vi "Conversao_todos_e_link_CLP.vi"() -> ()   [LabVIEW 2019]
uses:
  padrao_UCM.004.EEL.0300_ENTRADA.ctl
  padrao_UCM.004.EEL.0300_SAIDA.ctl
  padrao_UCM.004.EEL.0200_ENTRADA.ctl
  padrao_UCM.004.EEL.0200_SAIDA.ctl
  padrao_INTERNO.ctl
  padrao_todos_os_dados_ENTRADA.ctl
  padrao_todos_os_dados_SAIDA.ctl
  <vilib>/Utility/config.llb/NI_LVConfig.lvlib
panel:
  out "INTERNO":T1
  out "UCM.004.EEL.0200_ENTRADA_engenharia":T2
  out "X33-2":i16
  out "GD-ST-ES":i16
  out "X31-16":bool
  out "X31-15":bool
  out "X31-14":bool
  out "X31-13":bool
  out "X31-12":bool
  out "X31-11":bool
  out "X31-10":bool
  out "SHD-ON-OFF":bool
  out "SHD-CV-002":bool
  out "SHD-CV-001":bool
  out "SKS-CV-006":bool
  out "SKS-CV-005":bool
  out "SKS-CV-004":bool
  out "SKS-CV-003":bool
  out "SKS-CV-002":bool
  out "SKS-CV-001":bool
  in  "SIT-PI-03":i16
  in  "SIT-PI-MS3":i16
  in  "SHD-PI-02":i16
  in  "SHD-PI-01":i16
  in  "X32-4":i16
  in  "SHD-TI-AMB":i16
  in  "SKS-LC-W":i16
  in  "SKS-LC-K":i16
  in  "X30-16":bool
  in  "X30-15":bool
  in  "X30-14":bool
  in  "X30-13":bool
  in  "X30-12":bool
  in  "X30-11":bool
  in  "X30-10":bool
  in  "X30-9":bool
  in  "X30-8":bool
  in  "SKS-MAX-K":bool
  in  "SKS-MIN-K":bool
  in  "SKS-MAX-W":bool
  in  "SKS-MIN-W":bool
  in  "SKS-LAH-K":bool
  in  "SKS-LAH-W":bool
  in  "SKS-LAH-S":bool
  out "UCM.004.EEL.0200_SAIDA(%)":T3
  out "UCM.004.EEL.0200_SAIDA(Puro)":T3
  out "UCM.004.EEL.0200_ENTRADA_puro":T2
  out "UCM.004.EEL.0300_SAIDA(%)":T4
  in  "SKM-FIC-COR-AR":dbl
  out "PID-INV-KF-GD":dbl
  out "PID-INV-KF-GI":dbl
  out "PID-INV-KF-GP":dbl
  out "PID-INV-WF-GD":dbl
  out "PID-INV-WF-GI":dbl
  out "PID-INV-WF-GP":dbl
  out "PID-FC-KF-GD":dbl
  out "PID-FC-KF-GI":dbl
  out "PID-FC-KF-GP":dbl
  out "PID-FC-WF-GD":dbl
  out "PID-FC-WF-GI":dbl
  out "PID-FC-WF-GP":dbl
  out "PID-FC-AR-GD":dbl
  out "PID-FC-AR-GI":dbl
  out "PID-FC-AR-GP":dbl
  out "PID-PC-TQ-GD":dbl
  out "PID-PC-TQ-GI":dbl
  out "PID-PC-TQ-GP":dbl
  out "SKM-FIC-COR-KF-MIN":dbl
  out "SKM-FIC-COR-KF-MAX":dbl
  out "SKM-FIC-COR-AR-MIN":dbl
  out "SKM-FIC-COR-AR-MAX":dbl
  out "SPW-WR-VEL":i32
  out "SPK-WR-VEL":i32
  out "PID-INC-KF-SP":i16
  out "PID-INC-WF-SP":i16
  out "PID-FC-KF-SP":i16
  out "PID-FC-WF-SP":i16
  out "PID-FC-AR-SP":i16
  out "PID-PC-TQ-SP":i16
  out "X33 14":i16
  out "X33 13":i16
  out "X33 12":i16
  out "X33 11":i16
  out "X33 10":i16
  out "X33 9":i16
  out "X33 8":i16
  out "X33 7":i16
  out "X33 6":i16
  out "X33 5":i16
  out "SKM-FC-KF":i16
  out "SKM-FC-WF":i16
  out "SKM-FC-AR":i16
  out "SKM-PC-TQ":i16
  out "UCM.004.EEL.0300_SAIDA(Puro)":T4
  out "SPW-WR-OFF":bool
  out "SPK-WR-OFF":bool
  out "SPW-WR-ON":bool
  out "SPK-WR-ON":bool
  out "PID-SA-AR-COR":bool
  out "PID-SA-KF-INV":bool
  out "PID-SA-WF-INV":bool
  out "PID-KF-ON":bool
  out "PID-WF-ON":bool
  out "PID-FC-AR-ON":bool
  out "PID-PC-TQ-ON":bool
  out "X31-32":bool
  out "X31-31":bool
  out "X31-30":bool
  out "X31-29":bool
  out "X31-28":bool
  out "X31-27":bool
  out "SKI-CV-BY2":bool
  out "SKI-CV-ST":bool
  out "SKI-CV-WF-BY1":bool
  out "SKI-CV-WF-ST":bool
  out "SKI-CV-KF-BY1":bool
  out "SKI-CV-KF-ST":bool
  out "SKI-CV-AR":bool
  out "SKM-CV-JMP":bool
  out "SKM-CV-COR":bool
  out "SKM-CV-LAM":bool
  out "SPW-CV-008":bool
  out "SPW-CV-007":bool
  out "SPW-CV-006":bool
  out "SPW-CV-005":bool
  out "SPW-CV-004":bool
  out "SPW-CV-003":bool
  out "SPW-CV-002":bool
  out "SPW-CV-001":bool
  out "SPK-CV-008":bool
  out "SPK-CV-007":bool
  out "SPK-CV-006":bool
  out "SPK-CV-005":bool
  out "SPK-CV-004":bool
  out "SPK-CV-003":bool
  out "SPK-CV-002":bool
  out "SPK-CV-001":bool
  in  "SPW-RD-CRT":dbl
  in  "SPK-RD-CRT":dbl
  in  "SKM-DEN-COR-AR":dbl
  in  "SKM-TI-COR-AR":dbl
  in  "SKM-FIC-COR-KF":dbl
  in  "SKM-DEN-COR-KF":dbl
  in  "SKM-TI-COR-KF":dbl
  in  "SPW-RD-TU":i32
  in  "SPK-RD-TU":i32
  in  "SPW-RD-IA":i32
  in  "SPK-RD-IA":i32
  in  "SPW-RD-VEL":i32
  in  "SPK-RD-VEL":i32
  in  "SPW-RD-ST":i32
  in  "SPK-RD-ST":i32
  in  "X32 24":i16
  in  "X32 23":i16
  in  "X32 22":i16
  in  "X32 21":i16
  in  "X32 20":i16
  in  "X32 19":i16
  in  "X32 18":i16
  in  "X32 17":i16
  in  "X32 16":i16
  in  "SPK-PD-P":i16
  in  "SPW-PD-P":i16
  in  "SKM-TI-KF":i16
  in  "SIT-PI-MS2":i16
  in  "SIT-PI-MS1":i16
  in  "SKI-PD-ST":i16
  in  "SIT-PI-001":i16
  in  "SKM-FIM-WF":i16
  in  "SKM-TI-WF":i16
  in  "SKM-PD-LAM":i16
  in  "SKM-TI-LAM":i16
  in  "SKM-PA-LAM":i16
  in  "SKM-TI-TQ":i16
  in  "SKM-PA-TQ":i16
  in  "SKM-PA-BAR":i16
  in  "SPW-RD-FLL":bool
  in  "SPW-RD-VVT":bool
  in  "SPW-RD-ALR":bool
  in  "SPK-RD-FLL":bool
  in  "SPK-RD-VVT":bool
  in  "SPK-RD-ALR":bool
  in  "X30 16":bool
  in  "X30 15":bool
  in  "X30 14":bool
  in  "X30 13":bool
  in  "X30 12":bool
  in  "X30 11":bool
  in  "X30 10":bool
  in  "X30 9":bool
  in  "X30 8":bool
  in  "X30 7":bool
  in  "X30 6":bool
  in  "X30 5":bool
  in  "X30 4":bool
  in  "X30 3":bool
  in  "X30 2":bool
  in  "X30 1":bool
  out "UCM.004.EEL.0300_ENTRADA_engenharia":T5
  out "UCM.004.EEL.0300_ENTRADA_puro":T5
  in  "stop":bool
  # "DADOS INTERNO"
  # "LEITURA\nENTRADA"
  # "ESCRITA\nSAIDA"
  # "0300"
  # "0300"
  # "0200"
  # "0200"
  # "PURO"
  # "ENGENHARIA"
  # "PURO"
  # "ENGENHARIA"
  # "(%)"
  # "PURO"
  # "(%)"
  # "PURO"
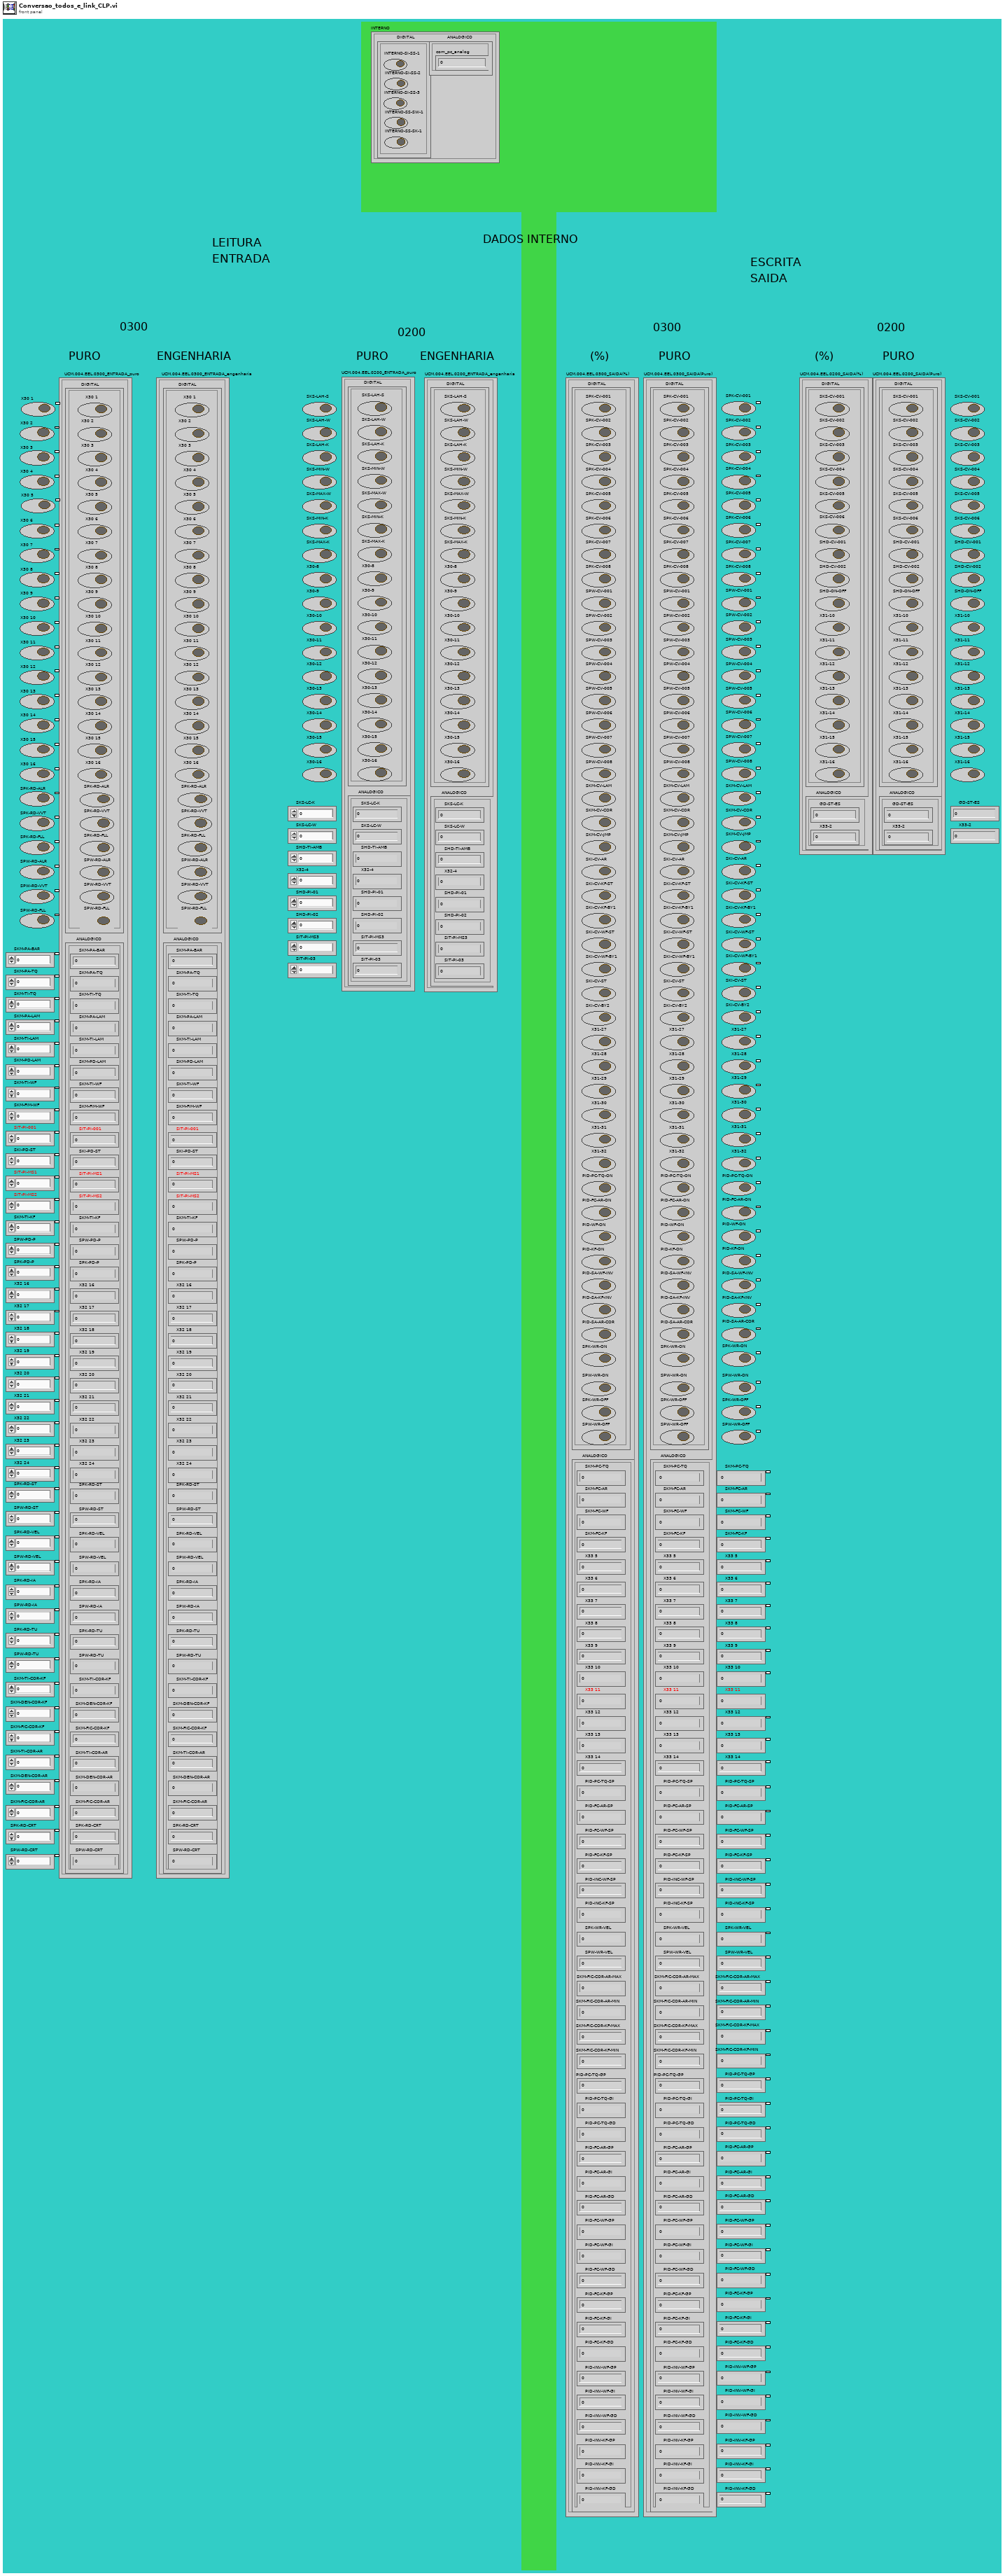
[diagram p1: front panel]
types:
  T1 = typedef "padrao_INTERNO.ctl" = cluster{"DIGITAL":cluster{"INTERNO-SI-SS-1":bool, "INTERNO-SI-SS-2":bool, "INTERNO-SI-SS-3":bool, "INTERNO-SS-SW-1":bool, "INTERNO-SS-SK-1":bool}, "ANALOGICO":cluster{"com_pc_analog":dbl}}
  T2 = typedef "padrao_UCM.004.EEL.0200_ENTRADA.ctl" = cluster{"DIGITAL":cluster{"SKS-LAH-S":bool, "SKS-LAH-W":bool, "SKS-LAH-K":bool, "SKS-MIN-W":bool, "SKS-MAX-W":bool, "SKS-MIN-K":bool, "SKS-MAX-K":bool, "X30-8":bool, "X30-9":bool, "X30-10":bool, "X30-11":bool, "X30-12":bool, "X30-13":bool, "X30-14":bool, "X30-15":bool, "X30-16":bool}, "ANALOGICO":cluster{"SKS-LC-K":i16, "SKS-LC-W":i16, "SHD-TI-AMB":i16, "X32-4":i16, "SHD-PI-01":i16, "SHD-PI-02":i16, "SIT-PI-MS3":i16, "SIT-PI-03":i16}}
  T3 = typedef "padrao_UCM.004.EEL.0200_SAIDA.ctl" = cluster{"DIGITAL":cluster{"SKS-CV-001":bool, "SKS-CV-002":bool, "SKS-CV-003":bool, "SKS-CV-004":bool, "SKS-CV-005":bool, "SKS-CV-006":bool, "SHD-CV-001":bool, "SHD-CV-002":bool, "SHD-ON-OFF":bool, "X31-10":bool, "X31-11":bool, "X31-12":bool, "X31-13":bool, "X31-14":bool, "X31-15":bool, "X31-16":bool}, "ANALOGICO":cluster{"GD-ST-ES":i16, "X33-2":i16}}
  T4 = typedef "padrao_UCM.004.EEL.0300_SAIDA.ctl" = cluster{"DIGITAL":cluster{"SPK-CV-001":bool, "SPK-CV-002":bool, "SPK-CV-003":bool, "SPK-CV-004":bool, "SPK-CV-005":bool, "SPK-CV-006":bool, "SPK-CV-007":bool, "SPK-CV-008":bool, "SPW-CV-001":bool, "SPW-CV-002":bool, "SPW-CV-003":bool, "SPW-CV-004":bool, "SPW-CV-005":bool, "SPW-CV-006":bool, "SPW-CV-007":bool, "SPW-CV-008":bool, "SKM-CV-LAM":bool, "SKM-CV-COR":bool, "SKM-CV-JMP":bool, "SKI-CV-AR":bool, "SKI-CV-KF-ST":bool, "SKI-CV-KF-BY1":bool, "SKI-CV-WF-ST":bool, "SKI-CV-WF-BY1":bool, "SKI-CV-ST":bool, "SKI-CV-BY2":bool, "X31-27":bool, "X31-28":bool, "X31-29":bool, "X31-30":bool, "X31-31":bool, "X31-32":bool, "PID-PC-TQ-ON":bool, "PID-FC-AR-ON":bool, "PID-WF-ON":bool, "PID-KF-ON":bool, "PID-SA-WF-INV":bool, "PID-SA-KF-INV":bool, "PID-SA-AR-COR":bool, "SPK-WR-ON":bool, "SPW-WR-ON":bool, "SPK-WR-OFF":bool, "SPW-WR-OFF":bool}, "ANALOGICO":cluster{"SKM-PC-TQ":i16, "SKM-FC-AR":i16, "SKM-FC-WF":i16, "SKM-FC-KF":i16, "X33 5":i16, "X33 6":i16, "X33 7":i16, "X33 8":i16, "X33 9":i16, "X33 10":i16, "X33 11":i16, "X33 12":i16, "X33 13":i16, "X33 14":i16, "PID-PC-TQ-SP":i16, "PID-FC-AR-SP":i16, "PID-FC-WF-SP":i16, "PID-FC-KF-SP":i16, "PID-INC-WF-SP":i16, "PID-INC-KF-SP":i16, "SPK-WR-VEL":i32, "SPW-WR-VEL":i32, "SKM-FIC-COR-AR-MAX":dbl, "SKM-FIC-COR-AR-MIN":dbl, "SKM-FIC-COR-KF-MAX":dbl, "SKM-FIC-COR-KF-MIN":dbl, "PID-PC-TQ-GP":dbl, "PID-PC-TQ-GI":dbl, "PID-PC-TQ-GD":dbl, "PID-FC-AR-GP":dbl, "PID-FC-AR-GI":dbl, "PID-FC-AR-GD":dbl, "PID-FC-WF-GP":dbl, "PID-FC-WF-GI":dbl, "PID-FC-WF-GD":dbl, "PID-FC-KF-GP":dbl, "PID-FC-KF-GI":dbl, "PID-FC-KF-GD":dbl, "PID-INV-WF-GP":dbl, "PID-INV-WF-GI":dbl, "PID-INV-WF-GD":dbl, "PID-INV-KF-GP":dbl, "PID-INV-KF-GI":dbl, "PID-INV-KF-GD":dbl}}
  T5 = typedef "padrao_UCM.004.EEL.0300_ENTRADA.ctl" = cluster{"DIGITAL":cluster{"X30 1":bool, "X30 2":bool, "X30 3":bool, "X30 4":bool, "X30 5":bool, "X30 6":bool, "X30 7":bool, "X30 8":bool, "X30 9":bool, "X30 10":bool, "X30 11":bool, "X30 12":bool, "X30 13":bool, "X30 14":bool, "X30 15":bool, "X30 16":bool, "SPK-RD-ALR":bool, "SPK-RD-VVT":bool, "SPK-RD-FLL":bool, "SPW-RD-ALR":bool, "SPW-RD-VVT":bool, "SPW-RD-FLL":bool}, "ANALOGICO":cluster{"SKM-PA-BAR":i16, "SKM-PA-TQ":i16, "SKM-TI-TQ":i16, "SKM-PA-LAM":i16, "SKM-TI-LAM":i16, "SKM-PD-LAM":i16, "SKM-TI-WF":i16, "SKM-FIM-WF":i16, "SIT-PI-001":i16, "SKI-PD-ST":i16, "SIT-PI-MS1":i16, "SIT-PI-MS2":i16, "SKM-TI-KF":i16, "SPW-PD-P":i16, "SPK-PD-P":i16, "X32 16 ":i16, "X32 17":i16, "X32 18":i16, "X32 19":i16, "X32 20":i16, "X32 21":i16, "X32 22":i16, "X32 23":i16, "X32 24":i16, "SPK-RD-ST":i32, "SPW-RD-ST":i32, "SPK-RD-VEL":i32, "SPW-RD-VEL":i32, "SPK-RD-IA":i32, "SPW-RD-IA":i32, "SPK-RD-TU":i32, "SPW-RD-TU":i32, "SKM-TI-COR-KF":dbl, "SKM-DEN-COR-KF":dbl, "SKM-FIC-COR-KF":dbl, "SKM-TI-COR-AR":dbl, "SKM-DEN-COR-AR":dbl, "SPK-RD-CRT":dbl, "SPW-RD-CRT":dbl, "SKM-FIC-COR-AR":dbl}}
  T6 = typedef "padrao_todos_os_dados_SAIDA.ctl" = cluster{"UCM.004.EEL.0300_SAIDA":T4, "UCM.004.EEL.0200_SAIDA":T3, "INTERNO":T1}
  T7 = typedef "padrao_todos_os_dados_ENTRADA.ctl" = cluster{"UCM.004.EEL.0300_ENTRADA":T5, "UCM.004.EEL.0200_ENTRADA":T2, "INTERNO":T1}
  T8 = typedef "NI_LVConfig.lvlib/Config Data RefNum.ctl" = refnum<k1>
  T9 = typedef "padrao_array_cluster_calibracao.ctl" = cluster{"TAG":string, "Minimo":dbl, "Fabricante":string, "Maximo":dbl, "remover_dipositvo":bool, "Modelo":string, "Numero de Serie":string}[]
  T10 = cluster{"SKS-CV-001":bool, "SKS-CV-002":bool, "SKS-CV-003":bool, "SKS-CV-004":bool, "SKS-CV-005":bool, "SKS-CV-006":bool, "SHD-CV-001":bool, "SHD-CV-002":bool, "SHD-ON-OFF":bool, "X31-10":bool, "X31-11":bool, "X31-12":bool, "X31-13":bool, "X31-14":bool, "X31-15":bool, "X31-16":bool}
  T11 = cluster{"SPK-CV-001":bool, "SPK-CV-002":bool, "SPK-CV-003":bool, "SPK-CV-004":bool, "SPK-CV-005":bool, "SPK-CV-006":bool, "SPK-CV-007":bool, "SPK-CV-008":bool, "SPW-CV-001":bool, "SPW-CV-002":bool, "SPW-CV-003":bool, "SPW-CV-004":bool, "SPW-CV-005":bool, "SPW-CV-006":bool, "SPW-CV-007":bool, "SPW-CV-008":bool, "SKM-CV-LAM":bool, "SKM-CV-COR":bool, "SKM-CV-JMP":bool, "SKI-CV-AR":bool, "SKI-CV-KF-ST":bool, "SKI-CV-KF-BY1":bool, "SKI-CV-WF-ST":bool, "SKI-CV-WF-BY1":bool, "SKI-CV-ST":bool, "SKI-CV-BY2":bool, "X31-27":bool, "X31-28":bool, "X31-29":bool, "X31-30":bool, "X31-31":bool, "X31-32":bool, "PID-PC-TQ-ON":bool, "PID-FC-AR-ON":bool, "PID-WF-ON":bool, "PID-KF-ON":bool, "PID-SA-WF-INV":bool, "PID-SA-KF-INV":bool, "PID-SA-AR-COR":bool, "SPK-WR-ON":bool, "SPW-WR-ON":bool, "SPK-WR-OFF":bool, "SPW-WR-OFF":bool}
  T12 = cluster{"SKM-PC-TQ":i16, "SKM-FC-AR":i16, "SKM-FC-WF":i16, "SKM-FC-KF":i16, "X33 5":i16, "X33 6":i16, "X33 7":i16, "X33 8":i16, "X33 9":i16, "X33 10":i16, "X33 11":i16, "X33 12":i16, "X33 13":i16, "X33 14":i16, "PID-PC-TQ-SP":i16, "PID-FC-AR-SP":i16, "PID-FC-WF-SP":i16, "PID-FC-KF-SP":i16, "PID-INC-WF-SP":i16, "PID-INC-KF-SP":i16, "SPK-WR-VEL":i32, "SPW-WR-VEL":i32, "SKM-FIC-COR-AR-MAX":dbl, "SKM-FIC-COR-AR-MIN":dbl, "SKM-FIC-COR-KF-MAX":dbl, "SKM-FIC-COR-KF-MIN":dbl, "PID-PC-TQ-GP":dbl, "PID-PC-TQ-GI":dbl, "PID-PC-TQ-GD":dbl, "PID-FC-AR-GP":dbl, "PID-FC-AR-GI":dbl, "PID-FC-AR-GD":dbl, "PID-FC-WF-GP":dbl, "PID-FC-WF-GI":dbl, "PID-FC-WF-GD":dbl, "PID-FC-KF-GP":dbl, "PID-FC-KF-GI":dbl, "PID-FC-KF-GD":dbl, "PID-INV-WF-GP":dbl, "PID-INV-WF-GI":dbl, "PID-INV-WF-GD":dbl, "PID-INV-KF-GP":dbl, "PID-INV-KF-GI":dbl, "PID-INV-KF-GD":dbl}
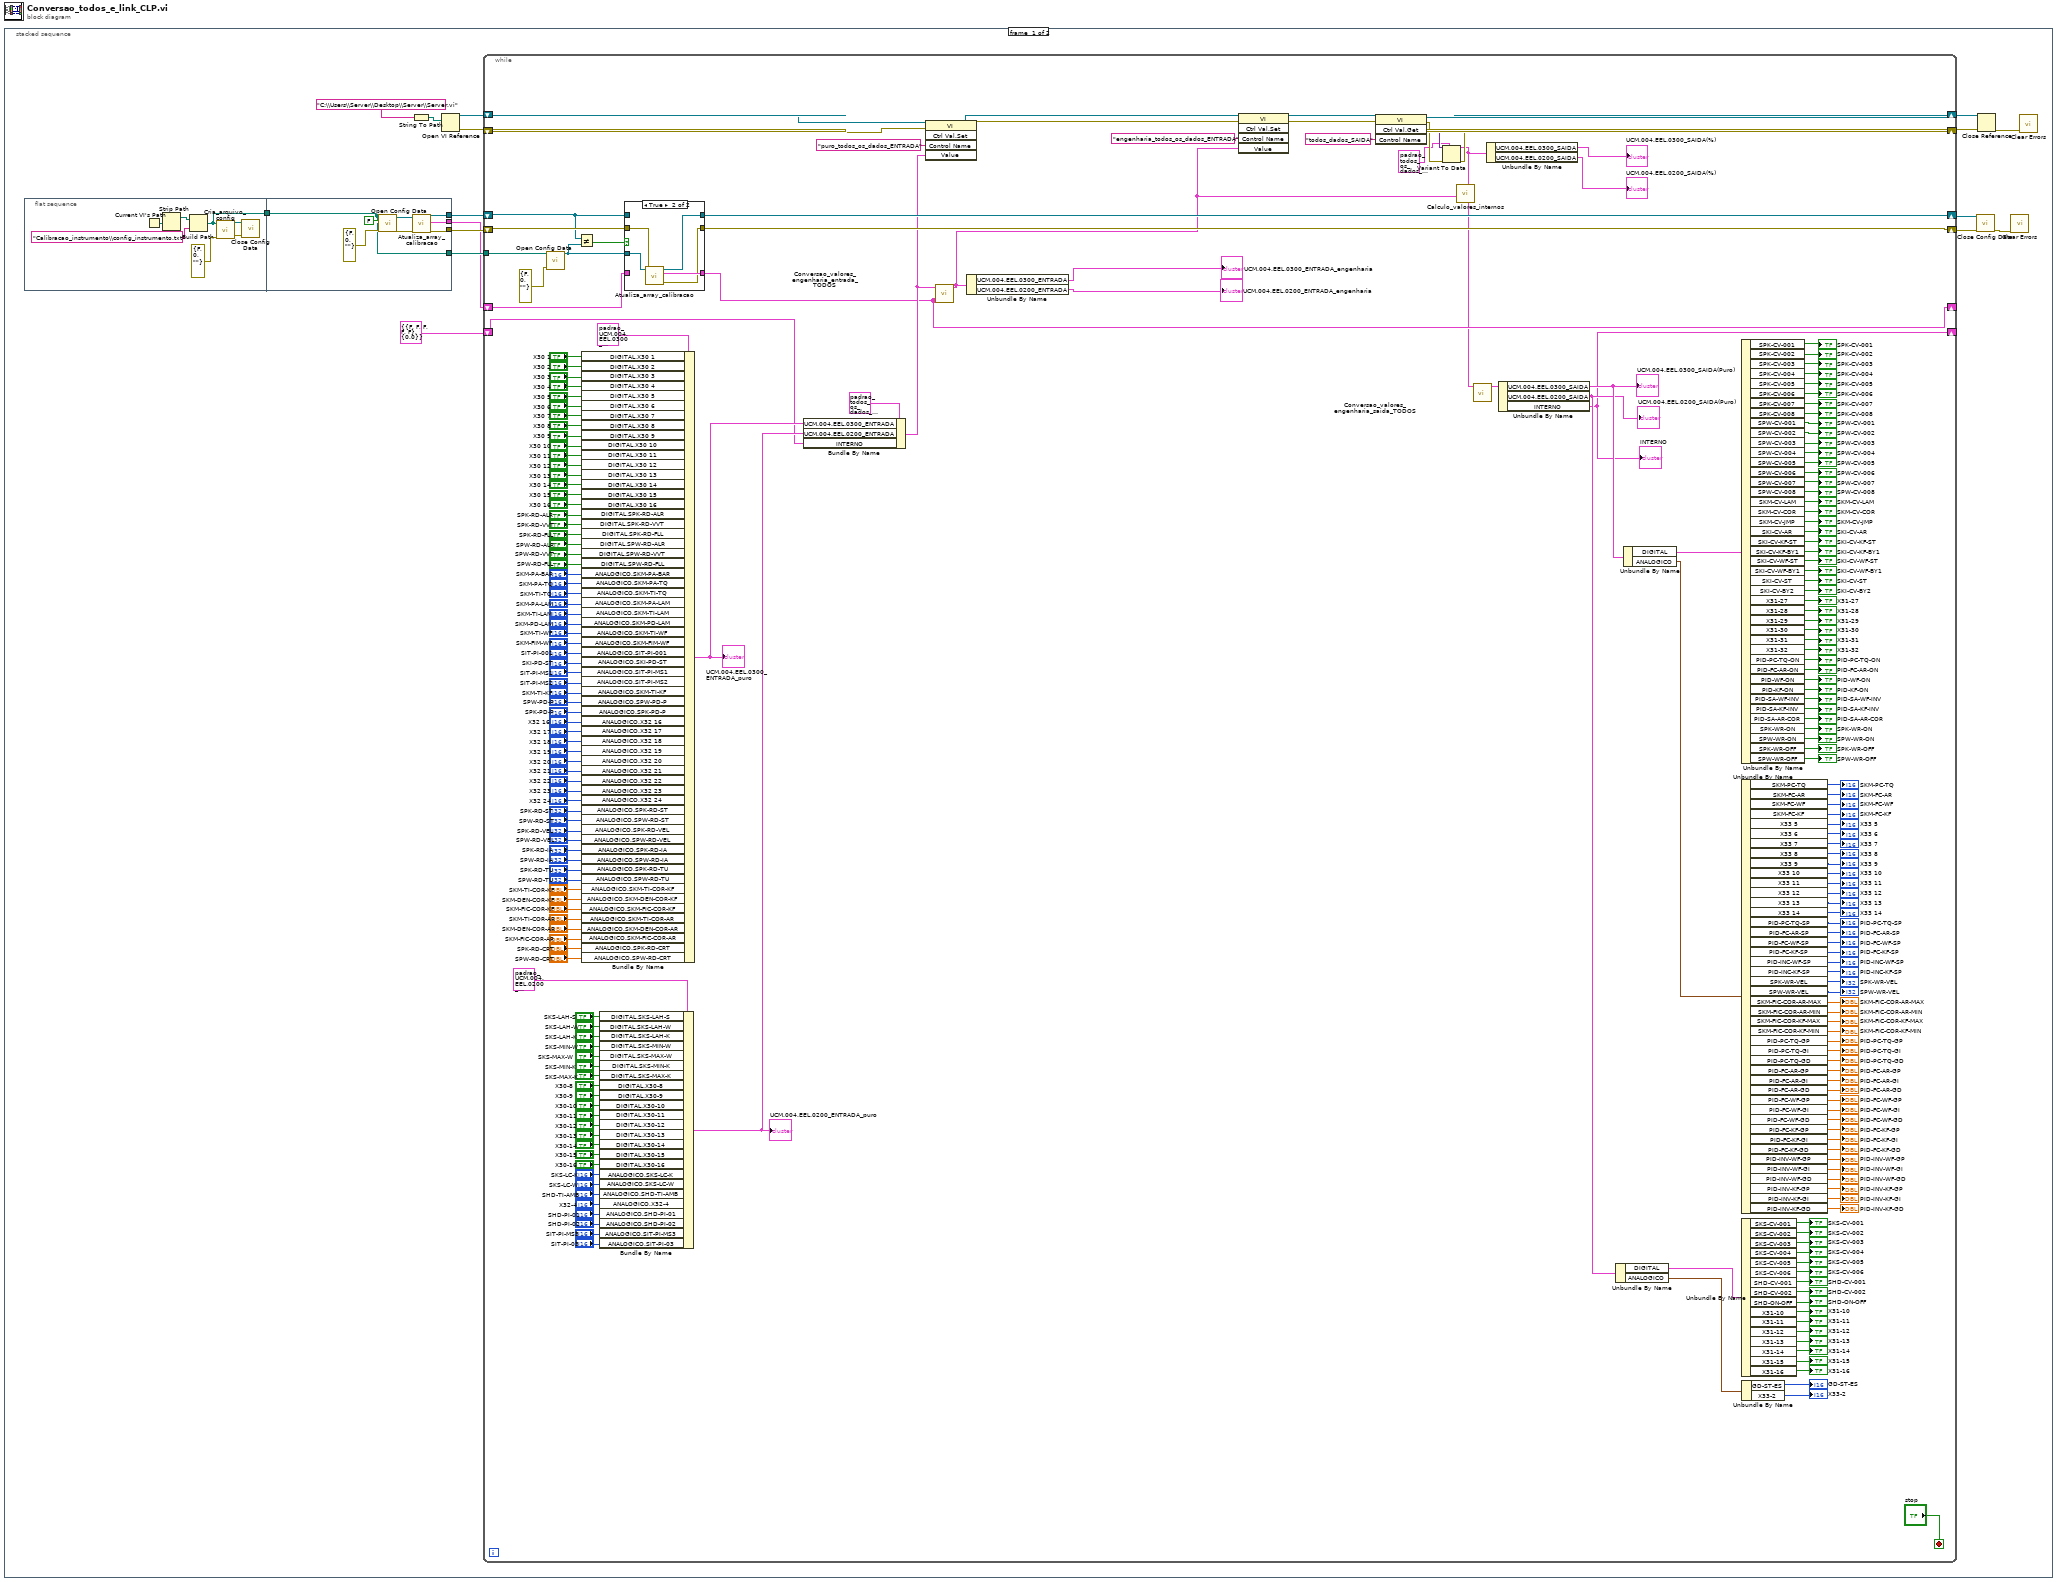
[diagram p0: block diagram]
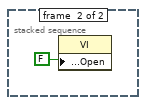
[diagram p3: hidden frame]
diagram:
  n1 = stacked-sequence {
    frame #0 {
      n2 = flat-sequence {
        tunnel: [w17] -> w6
        tunnel: w6 -> [w29]
        tunnel: [w28] -> w5
        tunnel: [w25] -> w4
        tunnel: [w29] -> w3
        tunnel: [w24] -> w2
        frame #0 {
          n3 = Current VI's Path() -> (path=w21:path)
          n4 = Strip Path(path=w21) -> (stripped path=w23:path)  [unwired: 1 out]
          n5 = Build Path(base path=w23, name or relative path="Calibracao_instrumento\\config_instrumento.txt") -> (appended path=w17:path)
          n6 = call "Cria_arquivo_config.vi"("error in (no error)"=errorcluster {"status"=FALSE, "code"=0, "source"=""}, "refnum in"=w17) -> ("error out"=w18:errorcluster, "refnum"=w19:T8)  [unwired: 8 in]
          n7 = call <vilib>:"Close Config Data.vi"("error in (no error)"=w18, "refnum"=w19) -> ()  [unwired: 8 in, 2 out]
        }
        frame #1 {
          n8 = call <vilib>:"Open Config Data.vi"("error in (no error)"=errorcluster {"status"=FALSE, "code"=0, "source"=""}, "create file if necessary (T)"=FALSE, "configuration file path"=w29) -> ("error out"=w26:errorcluster, "refnum"=w27:T8)  [unwired: 6 in, 1 out]
          n9 = call "Atualiza_array_calibracao.vi"("error in (no error)"=w26, "refnum"=w27) -> ("error out"=w25:errorcluster, "Instrumentos"=w24:T9, "refnum out"=w28:T8)  [unwired: 7 in]
        }
      }
      n10 = String To Path(string="C:\\Users\\Server\\Desktop\\Server\\Server.vi") -> (path=w15:path)
      n11 = Open VI Reference(vi path=w15) -> (vi reference=w13:refnum<vi>, error out=w14:errorcluster)  [unwired: 5 in]
      n12 = while {
        shift-right: [w258] -> w12
        shift-left: w13 -> [w269]
        shift-right: [w254] -> w11
        shift-left: w14 -> [w268]
        shift-right: [w98] -> w9
        shift-left: w5 -> [w94]
        shift-right: [w97] -> w8
        shift-left: w4 -> [w99]
        tunnel: w3 -> [w96]
        shift-right: [w86] -> _
        shift-left: w2 -> [w91]
        shift-right: [w35] -> _
        shift-left: T1 {"DIGITAL"={"INTERNO-SI-SS-1"=FALSE, "INTERNO-SI-SS-2"=FALSE, "INTERNO-SI-SS-3"=FALSE, "INTERNO-SS-SW-1"=FALSE, "INTERNO-SS-SK-1"=FALSE}, "ANALOGICO"={"com_pc_analog"=0.0}} ("INTERNO(Entrada)") -> [w36]
        stop <- "stop" stop-if-true
        n13 = call <vilib>:"Open Config Data.vi"("error in (no error)"=errorcluster {"status"=FALSE, "code"=0, "source"=""}, "configuration file path"=w96) -> ("refnum"=w92:T8)  [unwired: 7 in, 2 out]
        n14 = Not Equal?(x=w94, y=w92) -> (x != y?=w93:bool)
        n15 = Bundle By Name(cluster=T5 {"DIGITAL"={"X30 1"=FALSE, "X30 2"=FALSE, "X30 3"=FALSE, "X30 4"=FALSE, "X30 5"=FALSE, "X30 6"=FALSE, "X30 7"=FALSE, "X30 8"=FALSE, "X30 9"=FALSE, "X30 10"=FALSE, "X30 11"=FALSE, "X30 12"=FALSE, "X30 13"=FALSE, "X30 14"=FALSE, "X30 15"=FALSE, "X30 16"=FALSE, "SPK-RD-ALR"=FALSE, "SPK-RD-VVT"=FALSE, "SPK-RD-FLL"=FALSE, "SPW-RD-ALR"=FALSE, "SPW-RD-VVT"=FALSE, "SPW-RD-FLL"=FALSE}, "ANALOGICO"={"SKM-PA-BAR"=0, "SKM-PA-TQ"=0, "SKM-TI-TQ"=0, "SKM-PA-LAM"=0, "SKM-TI-LAM"=0, "SKM-PD-LAM"=0, "SKM-TI-WF"=0, "SKM-FIM-WF"=0, "SIT-PI-001"=0, "SKI-PD-ST"=0, "SIT-PI-MS1"=0, "SIT-PI-MS2"=0, "SKM-TI-KF"=0, "SPW-PD-P"=0, "SPK-PD-P"=0, "X32 16 "=0, "X32 17"=0, "X32 18"=0, "X32 19"=0, "X32 20"=0, "X32 21"=0, "X32 22"=0, "X32 23"=0, "X32 24"=0, "SPK-RD-ST"=0, "SPW-RD-ST"=0, "SPK-RD-VEL"=0, "SPW-RD-VEL"=0, "SPK-RD-IA"=0, "SPW-RD-IA"=0, "SPK-RD-TU"=0, "SPW-RD-TU"=0, "SKM-TI-COR-KF"=0.0, "SKM-DEN-COR-KF"=0.0, "SKM-FIC-COR-KF"=0.0, "SKM-TI-COR-AR"=0.0, "SKM-DEN-COR-AR"=0.0, "SPK-RD-CRT"=0.0, "SPW-RD-CRT"=0.0, "SKM-FIC-COR-AR"=0.0}} ("UCM.004.EEL.0300_ENTRADA_puro"), "DIGITAL.X30 1"="X30 1", "DIGITAL.X30 2"="X30 2", "DIGITAL.X30 3"="X30 3", "DIGITAL.X30 4"="X30 4", "DIGITAL.X30 5"="X30 5", "DIGITAL.X30 6"="X30 6", "DIGITAL.X30 7"="X30 7", "DIGITAL.X30 8"="X30 8", "DIGITAL.X30 9"="X30 9", "DIGITAL.X30 10"="X30 10", "DIGITAL.X30 11"="X30 11", "DIGITAL.X30 12"="X30 12", "DIGITAL.X30 13"="X30 13", "DIGITAL.X30 14"="X30 14", "DIGITAL.X30 15"="X30 15", "DIGITAL.X30 16"="X30 16", "DIGITAL.SPK-RD-ALR"="SPK-RD-ALR", "DIGITAL.SPK-RD-VVT"="SPK-RD-VVT", "DIGITAL.SPK-RD-FLL"="SPK-RD-FLL", "DIGITAL.SPW-RD-ALR"="SPW-RD-ALR", "DIGITAL.SPW-RD-VVT"="SPW-RD-VVT", "DIGITAL.SPW-RD-FLL"="SPW-RD-FLL", "ANALOGICO.SKM-PA-BAR"="SKM-PA-BAR", "ANALOGICO.SKM-PA-TQ"="SKM-PA-TQ", "ANALOGICO.SKM-TI-TQ"="SKM-TI-TQ", "ANALOGICO.SKM-PA-LAM"="SKM-PA-LAM", "ANALOGICO.SKM-TI-LAM"="SKM-TI-LAM", "ANALOGICO.SKM-PD-LAM"="SKM-PD-LAM", "ANALOGICO.SKM-TI-WF"="SKM-TI-WF", "ANALOGICO.SKM-FIM-WF"="SKM-FIM-WF", "ANALOGICO.SIT-PI-001"="SIT-PI-001", "ANALOGICO.SKI-PD-ST"="SKI-PD-ST", "ANALOGICO.SIT-PI-MS1"="SIT-PI-MS1", "ANALOGICO.SIT-PI-MS2"="SIT-PI-MS2", "ANALOGICO.SKM-TI-KF"="SKM-TI-KF", "ANALOGICO.SPW-PD-P"="SPW-PD-P", "ANALOGICO.SPK-PD-P"="SPK-PD-P", "ANALOGICO.X32 16"="X32 16", "ANALOGICO.X32 17"="X32 17", "ANALOGICO.X32 18"="X32 18", "ANALOGICO.X32 19"="X32 19", "ANALOGICO.X32 20"="X32 20", "ANALOGICO.X32 21"="X32 21", "ANALOGICO.X32 22"="X32 22", "ANALOGICO.X32 23"="X32 23", "ANALOGICO.X32 24"="X32 24", "ANALOGICO.SPK-RD-ST"="SPK-RD-ST", "ANALOGICO.SPW-RD-ST"="SPW-RD-ST", "ANALOGICO.SPK-RD-VEL"="SPK-RD-VEL", "ANALOGICO.SPW-RD-VEL"="SPW-RD-VEL", "ANALOGICO.SPK-RD-IA"="SPK-RD-IA", "ANALOGICO.SPW-RD-IA"="SPW-RD-IA", "ANALOGICO.SPK-RD-TU"="SPK-RD-TU", "ANALOGICO.SPW-RD-TU"="SPW-RD-TU", "ANALOGICO.SKM-TI-COR-KF"="SKM-TI-COR-KF", "ANALOGICO.SKM-DEN-COR-KF"="SKM-DEN-COR-KF", "ANALOGICO.SKM-FIC-COR-KF"="SKM-FIC-COR-KF", "ANALOGICO.SKM-TI-COR-AR"="SKM-TI-COR-AR", "ANALOGICO.SKM-DEN-COR-AR"="SKM-DEN-COR-AR", "ANALOGICO.SKM-FIC-COR-AR"="SKM-FIC-COR-AR", "ANALOGICO.SPK-RD-CRT"="SPK-RD-CRT", "ANALOGICO.SPW-RD-CRT"="SPW-RD-CRT") -> (w249:T5)
        "UCM.004.EEL.0300_ENTRADA_puro" <- w249
        n16 = Bundle By Name(cluster=T2 {"DIGITAL"={"SKS-LAH-S"=FALSE, "SKS-LAH-W"=FALSE, "SKS-LAH-K"=FALSE, "SKS-MIN-W"=FALSE, "SKS-MAX-W"=FALSE, "SKS-MIN-K"=FALSE, "SKS-MAX-K"=FALSE, "X30-8"=FALSE, "X30-9"=FALSE, "X30-10"=FALSE, "X30-11"=FALSE, "X30-12"=FALSE, "X30-13"=FALSE, "X30-14"=FALSE, "X30-15"=FALSE, "X30-16"=FALSE}, "ANALOGICO"={"SKS-LC-K"=0, "SKS-LC-W"=0, "SHD-TI-AMB"=0, "X32-4"=0, "SHD-PI-01"=0, "SHD-PI-02"=0, "SIT-PI-MS3"=0, "SIT-PI-03"=0}} ("UCM.004.EEL.0200_ENTRADA"), "DIGITAL.SKS-LAH-S"="SKS-LAH-S", "DIGITAL.SKS-LAH-W"="SKS-LAH-W", "DIGITAL.SKS-LAH-K"="SKS-LAH-K", "DIGITAL.SKS-MIN-W"="SKS-MIN-W", "DIGITAL.SKS-MAX-W"="SKS-MAX-W", "DIGITAL.SKS-MIN-K"="SKS-MIN-K", "DIGITAL.SKS-MAX-K"="SKS-MAX-K", "DIGITAL.X30-8"="X30-8", "DIGITAL.X30-9"="X30-9", "DIGITAL.X30-10"="X30-10", "DIGITAL.X30-11"="X30-11", "DIGITAL.X30-12"="X30-12", "DIGITAL.X30-13"="X30-13", "DIGITAL.X30-14"="X30-14", "DIGITAL.X30-15"="X30-15", "DIGITAL.X30-16"="X30-16", "ANALOGICO.SKS-LC-K"="SKS-LC-K", "ANALOGICO.SKS-LC-W"="SKS-LC-W", "ANALOGICO.SHD-TI-AMB"="SHD-TI-AMB", "ANALOGICO.X32-4"="X32-4", "ANALOGICO.SHD-PI-01"="SHD-PI-01", "ANALOGICO.SHD-PI-02"="SHD-PI-02", "ANALOGICO.SIT-PI-MS3"="SIT-PI-MS3", "ANALOGICO.SIT-PI-03"="SIT-PI-03") -> (w84:T2)
        "UCM.004.EEL.0200_ENTRADA_puro" <- w84
        n17 = case shown="True" w93 {
          tunnel: [w270 w277] -> w86
          tunnel: w99 -> [w271 w276]
          tunnel: [w272 w275] -> w98
          tunnel: [w271 w274] -> w97
          tunnel: w94 -> [w272 _]
          tunnel: w92 -> [_ w273]
          tunnel: w91 -> [w270 _]
          frame False {
          }
          frame True {
            n18 = call "Atualiza_array_calibracao.vi"("error in (no error)"=w276, "refnum"=w273) -> ("error out"=w274:errorcluster, "Instrumentos"=w277:T9, "refnum out"=w275:T8)  [unwired: 7 in]
          }
        }
        n19 = Bundle By Name(cluster=T7 {"UCM.004.EEL.0300_ENTRADA"={"DIGITAL"={"X30 1"=FALSE, "X30 2"=FALSE, "X30 3"=FALSE, "X30 4"=FALSE, "X30 5"=FALSE, "X30 6"=FALSE, "X30 7"=FALSE, "X30 8"=FALSE, "X30 9"=FALSE, "X30 10"=FALSE, "X30 11"=FALSE, "X30 12"=FALSE, "X30 13"=FALSE, "X30 14"=FALSE, "X30 15"=FALSE, "X30 16"=FALSE, "SPK-RD-ALR"=FALSE, "SPK-RD-VVT"=FALSE, "SPK-RD-FLL"=FALSE, "SPW-RD-ALR"=FALSE, "SPW-RD-VVT"=FALSE, "SPW-RD-FLL"=FALSE}, "ANALOGICO"={"SKM-PA-BAR"=0, "SKM-PA-TQ"=0, "SKM-TI-TQ"=0, "SKM-PA-LAM"=0, "SKM-TI-LAM"=0, "SKM-PD-LAM"=0, "SKM-TI-WF"=0, "SKM-FIM-WF"=0, "SIT-PI-001"=0, "SKI-PD-ST"=0, "SIT-PI-MS1"=0, "SIT-PI-MS2"=0, "SKM-TI-KF"=0, "SPW-PD-P"=0, "SPK-PD-P"=0, "X32 16 "=0, "X32 17"=0, "X32 18"=0, "X32 19"=0, "X32 20"=0, "X32 21"=0, "X32 22"=0, "X32 23"=0, "X32 24"=0, "SPK-RD-ST"=0, "SPW-RD-ST"=0, "SPK-RD-VEL"=0, "SPW-RD-VEL"=0, "SPK-RD-IA"=0, "SPW-RD-IA"=0, "SPK-RD-TU"=0, "SPW-RD-TU"=0, "SKM-TI-COR-KF"=0.0, "SKM-DEN-COR-KF"=0.0, "SKM-FIC-COR-KF"=0.0, "SKM-TI-COR-AR"=0.0, "SKM-DEN-COR-AR"=0.0, "SPK-RD-CRT"=0.0, "SPW-RD-CRT"=0.0, "SKM-FIC-COR-AR"=0.0}}, "UCM.004.EEL.0200_ENTRADA"={"DIGITAL"={"SKS-LAH-S"=FALSE, "SKS-LAH-W"=FALSE, "SKS-LAH-K"=FALSE, "SKS-MIN-W"=FALSE, "SKS-MAX-W"=FALSE, "SKS-MIN-K"=FALSE, "SKS-MAX-K"=FALSE, "X30-8"=FALSE, "X30-9"=FALSE, "X30-10"=FALSE, "X30-11"=FALSE, "X30-12"=FALSE, "X30-13"=FALSE, "X30-14"=FALSE, "X30-15"=FALSE, "X30-16"=FALSE}, "ANALOGICO"={"SKS-LC-K"=0, "SKS-LC-W"=0, "SHD-TI-AMB"=0, "X32-4"=0, "SHD-PI-01"=0, "SHD-PI-02"=0, "SIT-PI-MS3"=0, "SIT-PI-03"=0}}, "INTERNO"={"DIGITAL"={"INTERNO-SI-SS-1"=FALSE, "INTERNO-SI-SS-2"=FALSE, "INTERNO-SI-SS-3"=FALSE, "INTERNO-SS-SW-1"=FALSE, "INTERNO-SS-SK-1"=FALSE}, "ANALOGICO"={"com_pc_analog"=0.0}}} ("todos_os_dados_ENTRADA"), "UCM.004.EEL.0300_ENTRADA"=w249, "UCM.004.EEL.0200_ENTRADA"=w84, "INTERNO"=w36) -> (w90:T7)
        n20 = invoke class="VI" method="Ctrl Val.Set"(reference=w269, error in=w268, "Control Name"="puro_todos_os_dados_ENTRADA", "Value"=w90) -> (reference out=w267:refnum<vi>, error out=w266:errorcluster)  [unwired: 1 in, 3 out]
        n21 = call "Conversao_valores_engenharia_entrada_TODOS.vi"("Instrumentos"=w86, "todos_os_dados_ENTRADA(Controle)"=w90) -> ("todos_os_dados_ENTRADA(Indicador)"=w34:T7)  [unwired: 5 in]
        n22 = Unbundle By Name(w34) -> ("UCM.004.EEL.0300_ENTRADA"=→"UCM.004.EEL.0300_ENTRADA_engenharia":T5, "UCM.004.EEL.0200_ENTRADA"=→"UCM.004.EEL.0200_ENTRADA_engenharia":T2)
        n23 = invoke class="VI" method="Ctrl Val.Set"(reference=w267, error in=w266, "Control Name"="engenharia_todos_os_dados_ENTRADA", "Value"=w34) -> (reference out=w260:refnum<vi>, error out=w259:errorcluster)  [unwired: 1 in, 3 out]
        n24 = invoke class="VI" method="Ctrl Val.Get"(reference=w260, error in=w259, "Control Name"="todos_dados_SAIDA") -> (reference out=w258:refnum<vi>, error out=w255:errorcluster, "Get Control Value Variant"=w256:variant)  [unwired: 1 in, 1 out]
        n25 = Variant To Data(error in=w255, type=T6 {"UCM.004.EEL.0300_SAIDA"={"DIGITAL"={"SPK-CV-001"=FALSE, "SPK-CV-002"=FALSE, "SPK-CV-003"=FALSE, "SPK-CV-004"=FALSE, "SPK-CV-005"=FALSE, "SPK-CV-006"=FALSE, "SPK-CV-007"=FALSE, "SPK-CV-008"=FALSE, "SPW-CV-001"=FALSE, "SPW-CV-002"=FALSE, "SPW-CV-003"=FALSE, "SPW-CV-004"=FALSE, "SPW-CV-005"=FALSE, "SPW-CV-006"=FALSE, "SPW-CV-007"=FALSE, "SPW-CV-008"=FALSE, "SKM-CV-LAM"=FALSE, "SKM-CV-COR"=FALSE, "SKM-CV-JMP"=FALSE, "SKI-CV-AR"=FALSE, "SKI-CV-KF-ST"=FALSE, "SKI-CV-KF-BY1"=FALSE, "SKI-CV-WF-ST"=FALSE, "SKI-CV-WF-BY1"=FALSE, "SKI-CV-ST"=FALSE, "SKI-CV-BY2"=FALSE, "X31-27"=FALSE, "X31-28"=FALSE, "X31-29"=FALSE, "X31-30"=FALSE, "X31-31"=FALSE, "X31-32"=FALSE, "PID-PC-TQ-ON"=FALSE, "PID-FC-AR-ON"=FALSE, "PID-WF-ON"=FALSE, "PID-KF-ON"=FALSE, "PID-SA-WF-INV"=FALSE, "PID-SA-KF-INV"=FALSE, "PID-SA-AR-COR"=FALSE, "SPK-WR-ON"=FALSE, "SPW-WR-ON"=FALSE, "SPK-WR-OFF"=FALSE, "SPW-WR-OFF"=FALSE}, "ANALOGICO"={"SKM-PC-TQ"=0, "SKM-FC-AR"=0, "SKM-FC-WF"=0, "SKM-FC-KF"=0, "X33 5"=0, "X33 6"=0, "X33 7"=0, "X33 8"=0, "X33 9"=0, "X33 10"=0, "X33 11"=0, "X33 12"=0, "X33 13"=0, "X33 14"=0, "PID-PC-TQ-SP"=0, "PID-FC-AR-SP"=0, "PID-FC-WF-SP"=0, "PID-FC-KF-SP"=0, "PID-INC-WF-SP"=0, "PID-INC-KF-SP"=0, "SPK-WR-VEL"=0, "SPW-WR-VEL"=0, "SKM-FIC-COR-AR-MAX"=0.0, "SKM-FIC-COR-AR-MIN"=0.0, "SKM-FIC-COR-KF-MAX"=0.0, "SKM-FIC-COR-KF-MIN"=0.0, "PID-PC-TQ-GP"=0.0, "PID-PC-TQ-GI"=0.0, "PID-PC-TQ-GD"=0.0, "PID-FC-AR-GP"=0.0, "PID-FC-AR-GI"=0.0, "PID-FC-AR-GD"=0.0, "PID-FC-WF-GP"=0.0, "PID-FC-WF-GI"=0.0, "PID-FC-WF-GD"=0.0, "PID-FC-KF-GP"=0.0, "PID-FC-KF-GI"=0.0, "PID-FC-KF-GD"=0.0, "PID-INV-WF-GP"=0.0, "PID-INV-WF-GI"=0.0, "PID-INV-WF-GD"=0.0, "PID-INV-KF-GP"=0.0, "PID-INV-KF-GI"=0.0, "PID-INV-KF-GD"=0.0}}, "UCM.004.EEL.0200_SAIDA"={"DIGITAL"={"SKS-CV-001"=FALSE, "SKS-CV-002"=FALSE, "SKS-CV-003"=FALSE, "SKS-CV-004"=FALSE, "SKS-CV-005"=FALSE, "SKS-CV-006"=FALSE, "SHD-CV-001"=FALSE, "SHD-CV-002"=FALSE, "SHD-ON-OFF"=FALSE, "X31-10"=FALSE, "X31-11"=FALSE, "X31-12"=FALSE, "X31-13"=FALSE, "X31-14"=FALSE, "X31-15"=FALSE, "X31-16"=FALSE}, "ANALOGICO"={"GD-ST-ES"=0, "X33-2"=0}}, "INTERNO"={"DIGITAL"={"INTERNO-SI-SS-1"=FALSE, "INTERNO-SI-SS-2"=FALSE, "INTERNO-SI-SS-3"=FALSE, "INTERNO-SS-SW-1"=FALSE, "INTERNO-SS-SK-1"=FALSE}, "ANALOGICO"={"com_pc_analog"=0.0}}} ("todos_os_dados_SAIDA"), Variant=w256) -> (data=w33:T6, error out=w254:errorcluster)
        n26 = call "Calculo_valores_internos.vi"("todos_os_dados_ENTRADA(engenharia)"=w34, "todos_dados_SAIDA(controle)"=w33) -> ("todos_dados_SAIDA"=w32:T6)  [unwired: 8 in]
        n27 = call "Conversao_valores_engenharia_saida_TODOS.vi"("todos_os_dados_SAIDA(Controle)"=w32) -> ("todos_os_dados_SAIDA(Indicador)"=w89:T6)  [unwired: 10 in]
        n28 = Unbundle By Name(w33) -> ("UCM.004.EEL.0300_SAIDA"=→"UCM.004.EEL.0300_SAIDA(%)":T4, "UCM.004.EEL.0200_SAIDA"=→"UCM.004.EEL.0200_SAIDA(%)":T3)
        n29 = Unbundle By Name(w89) -> ("UCM.004.EEL.0300_SAIDA"=w88:T4, "UCM.004.EEL.0200_SAIDA"=w82:T3, "INTERNO"=w35:T1)
        "UCM.004.EEL.0300_SAIDA(Puro)" <- w88
        "UCM.004.EEL.0200_SAIDA(Puro)" <- w82
        "INTERNO" <- w35
        n30 = Unbundle By Name(w82) -> ("DIGITAL"=w81:T10, "ANALOGICO"=w80:cluster{"GD-ST-ES":i16, "X33-2":i16})
        n31 = Unbundle By Name(w88) -> ("DIGITAL"=w252:T11, "ANALOGICO"=w251:T12)
        n32 = Unbundle By Name(w252) -> ("SPK-CV-001"=→"SPK-CV-001":bool, "SPK-CV-002"=→"SPK-CV-002":bool, "SPK-CV-003"=→"SPK-CV-003":bool, "SPK-CV-004"=→"SPK-CV-004":bool, "SPK-CV-005"=→"SPK-CV-005":bool, "SPK-CV-006"=→"SPK-CV-006":bool, "SPK-CV-007"=→"SPK-CV-007":bool, "SPK-CV-008"=→"SPK-CV-008":bool, "SPW-CV-001"=→"SPW-CV-001":bool, "SPW-CV-002"=→"SPW-CV-002":bool, "SPW-CV-003"=→"SPW-CV-003":bool, "SPW-CV-004"=→"SPW-CV-004":bool, "SPW-CV-005"=→"SPW-CV-005":bool, "SPW-CV-006"=→"SPW-CV-006":bool, "SPW-CV-007"=→"SPW-CV-007":bool, "SPW-CV-008"=→"SPW-CV-008":bool, "SKM-CV-LAM"=→"SKM-CV-LAM":bool, "SKM-CV-COR"=→"SKM-CV-COR":bool, "SKM-CV-JMP"=→"SKM-CV-JMP":bool, "SKI-CV-AR"=→"SKI-CV-AR":bool, "SKI-CV-KF-ST"=→"SKI-CV-KF-ST":bool, "SKI-CV-KF-BY1"=→"SKI-CV-KF-BY1":bool, "SKI-CV-WF-ST"=→"SKI-CV-WF-ST":bool, "SKI-CV-WF-BY1"=→"SKI-CV-WF-BY1":bool, "SKI-CV-ST"=→"SKI-CV-ST":bool, "SKI-CV-BY2"=→"SKI-CV-BY2":bool, "X31-27"=→"X31-27":bool, "X31-28"=→"X31-28":bool, "X31-29"=→"X31-29":bool, "X31-30"=→"X31-30":bool, "X31-31"=→"X31-31":bool, "X31-32"=→"X31-32":bool, "PID-PC-TQ-ON"=→"PID-PC-TQ-ON":bool, "PID-FC-AR-ON"=→"PID-FC-AR-ON":bool, "PID-WF-ON"=→"PID-WF-ON":bool, "PID-KF-ON"=→"PID-KF-ON":bool, "PID-SA-WF-INV"=→"PID-SA-WF-INV":bool, "PID-SA-KF-INV"=→"PID-SA-KF-INV":bool, "PID-SA-AR-COR"=→"PID-SA-AR-COR":bool, "SPK-WR-ON"=→"SPK-WR-ON":bool, "SPW-WR-ON"=→"SPW-WR-ON":bool, "SPK-WR-OFF"=→"SPK-WR-OFF":bool, "SPW-WR-OFF"=→"SPW-WR-OFF":bool)
        n33 = Unbundle By Name(w251) -> ("SKM-PC-TQ"=→"SKM-PC-TQ":i16, "SKM-FC-AR"=→"SKM-FC-AR":i16, "SKM-FC-WF"=→"SKM-FC-WF":i16, "SKM-FC-KF"=→"SKM-FC-KF":i16, "X33 5"=→"X33 5":i16, "X33 6"=→"X33 6":i16, "X33 7"=→"X33 7":i16, "X33 8"=→"X33 8":i16, "X33 9"=→"X33 9":i16, "X33 10"=→"X33 10":i16, "X33 11"=→"X33 11":i16, "X33 12"=→"X33 12":i16, "X33 13"=→"X33 13":i16, "X33 14"=→"X33 14":i16, "PID-PC-TQ-SP"=→"PID-PC-TQ-SP":i16, "PID-FC-AR-SP"=→"PID-FC-AR-SP":i16, "PID-FC-WF-SP"=→"PID-FC-WF-SP":i16, "PID-FC-KF-SP"=→"PID-FC-KF-SP":i16, "PID-INC-WF-SP"=→"PID-INC-WF-SP":i16, "PID-INC-KF-SP"=→"PID-INC-KF-SP":i16, "SPK-WR-VEL"=→"SPK-WR-VEL":i32, "SPW-WR-VEL"=→"SPW-WR-VEL":i32, "SKM-FIC-COR-AR-MAX"=→"SKM-FIC-COR-AR-MAX":dbl, "SKM-FIC-COR-AR-MIN"=→"SKM-FIC-COR-AR-MIN":dbl, "SKM-FIC-COR-KF-MAX"=→"SKM-FIC-COR-KF-MAX":dbl, "SKM-FIC-COR-KF-MIN"=→"SKM-FIC-COR-KF-MIN":dbl, "PID-PC-TQ-GP"=→"PID-PC-TQ-GP":dbl, "PID-PC-TQ-GI"=→"PID-PC-TQ-GI":dbl, "PID-PC-TQ-GD"=→"PID-PC-TQ-GD":dbl, "PID-FC-AR-GP"=→"PID-FC-AR-GP":dbl, "PID-FC-AR-GI"=→"PID-FC-AR-GI":dbl, "PID-FC-AR-GD"=→"PID-FC-AR-GD":dbl, "PID-FC-WF-GP"=→"PID-FC-WF-GP":dbl, "PID-FC-WF-GI"=→"PID-FC-WF-GI":dbl, "PID-FC-WF-GD"=→"PID-FC-WF-GD":dbl, "PID-FC-KF-GP"=→"PID-FC-KF-GP":dbl, "PID-FC-KF-GI"=→"PID-FC-KF-GI":dbl, "PID-FC-KF-GD"=→"PID-FC-KF-GD":dbl, "PID-INV-WF-GP"=→"PID-INV-WF-GP":dbl, "PID-INV-WF-GI"=→"PID-INV-WF-GI":dbl, "PID-INV-WF-GD"=→"PID-INV-WF-GD":dbl, "PID-INV-KF-GP"=→"PID-INV-KF-GP":dbl, "PID-INV-KF-GI"=→"PID-INV-KF-GI":dbl, "PID-INV-KF-GD"=→"PID-INV-KF-GD":dbl)
        n34 = Unbundle By Name(w81) -> ("SKS-CV-001"=→"SKS-CV-001":bool, "SKS-CV-002"=→"SKS-CV-002":bool, "SKS-CV-003"=→"SKS-CV-003":bool, "SKS-CV-004"=→"SKS-CV-004":bool, "SKS-CV-005"=→"SKS-CV-005":bool, "SKS-CV-006"=→"SKS-CV-006":bool, "SHD-CV-001"=→"SHD-CV-001":bool, "SHD-CV-002"=→"SHD-CV-002":bool, "SHD-ON-OFF"=→"SHD-ON-OFF":bool, "X31-10"=→"X31-10":bool, "X31-11"=→"X31-11":bool, "X31-12"=→"X31-12":bool, "X31-13"=→"X31-13":bool, "X31-14"=→"X31-14":bool, "X31-15"=→"X31-15":bool, "X31-16"=→"X31-16":bool)
        n35 = Unbundle By Name(w80) -> ("GD-ST-ES"=→"GD-ST-ES":i16, "X33-2"=→"X33-2":i16)
      }
      n36 = call <vilib>:"Close Config Data.vi"("error in (no error)"=w8, "refnum"=w9) -> ("error out"=w7:errorcluster)  [unwired: 8 in, 1 out]
      n37 = Close Reference(reference=w12, error in (no error)=w11) -> (error out=w10:errorcluster)
      n38 = call <vilib>:"Clear Errors.vi"("error in (no error)"=w7) -> ()  [unwired: 5 in, 2 out]
      n39 = call <vilib>:"Clear Errors.vi"("error in (no error)"=w10) -> ()  [unwired: 5 in, 2 out]
    }
    frame #1 {
      n40 = property class="VI"("Front Panel.Open"=FALSE ("Front Panel Window:Open")) -> ()  [unwired: 2 in, 2 out]
    }
  }
